vi "BfrPkt - Add Channels.vi"(8 "error in (no error)":errorcluster, 11 "Node Ptr":T1 format="%.0x") -> (0 "error out":errorcluster, 3 "Node Ptr out":T1 format="%.0x")   [LabVIEW 2016, in "UDP-Custom-Device System Explorer.lvlib"]
uses:
  UDP-Custom-Device System Explorer.lvlib
  <vilib>/NI Veristand/Custom Device API/Custom Device Item Ref.ctl
  <vilib>/NI Veristand/Custom Device API/Custom Device Channel.ctl
  <vilib>/NI Veristand/Custom Device API/Custom Device Channel Type.ctl
  <vilib>/NI VeriStand/Custom Device API/Custom Device API.lvlib
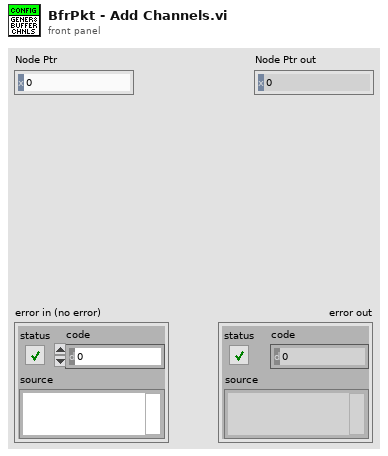
[diagram p1: front panel]
types:
  T1 = typedef "Custom Device API.lvlib/Custom Device Item Ref.ctl" = u64
  T2 = typedef "Custom Device API.lvlib/Custom Device Channel.ctl" = cluster{"Type":T3, "Units":string, "Default Value":dbl, "Faultable":bool, "Scalable":bool}
  T3 = typedef "Custom Device API.lvlib/Custom Device Channel Type.ctl" = enum16{"Input", "Output"}
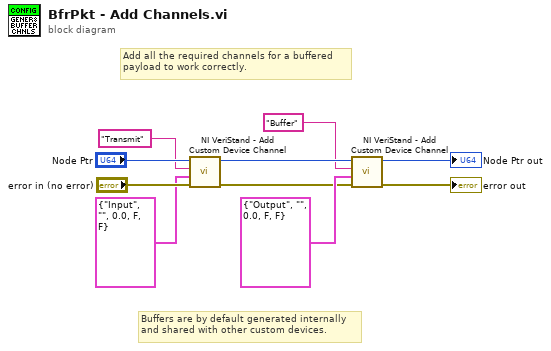
[diagram p0: block diagram]
diagram:
  # "Buffers are by default generated internally\nand shared with other custom devices."
  # "Add all the required channels for a buffered\npayload to work correctly."
  n1 = call <vilib>:"NI VeriStand - Add Custom Device Channel.vi"("error in (no error)"="error in (no error)", "Channel"=T2 {"Type"=enum."Input", "Units"="", "Default Value"=0.0, "Faultable"=FALSE, "Scalable"=FALSE}, "Channel Name"="Transmit", "Parent Ref in"="Node Ptr") -> ("error out"=w3:errorcluster, "Parent Ref out"=w6:T1)  [unwired: 4 in, 2 out]
  n2 = call <vilib>:"NI VeriStand - Add Custom Device Channel.vi"("error in (no error)"=w3, "Channel"=T2 {"Type"=enum."Output", "Units"="", "Default Value"=0.0, "Faultable"=FALSE, "Scalable"=FALSE}, "Channel Name"="Buffer", "Parent Ref in"=w6) -> ("error out"=→"error out":errorcluster, "Parent Ref out"=→"Node Ptr out":T1)  [unwired: 4 in, 2 out]
